vi "Create_Error.vi"(6 "Call chain":string[](array[string]), 7 "Restart text (\"\")":string, 8 "Status/Errors in":refnum<vi>, 9 "HiSPARC error":string, 10 "Warning? (false)":bool, 11 "Master?":T1) -> (0 "Status/Errors out":refnum<vi>)   [LabVIEW 2010]
doc: "Updates the Status/Errors-cluster with the message given by \"HiSPARC error\" together with the current time."
uses:
  Controls/Master.ctl
  Controls/Status_Errors_Elements.ctl
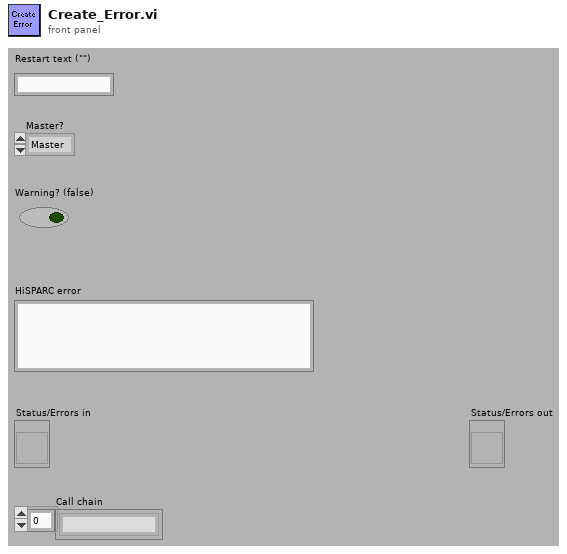
[diagram p1: front panel]
types:
  T1 = typedef "Master.ctl" = enum16{"Master", "Slave", "General"}
  T2 = typedef "Status_Errors_Elements.ctl" = enum16{"Default", "Errors", "Master status", "Slave status", "Master connected?", "Slave connected?", "Master GPS on board?", "Slave GPS on board?", "Master: slave detected?", "Slave: slave detected?", "Last message from master", "Last message from slave", "Master temperature"}
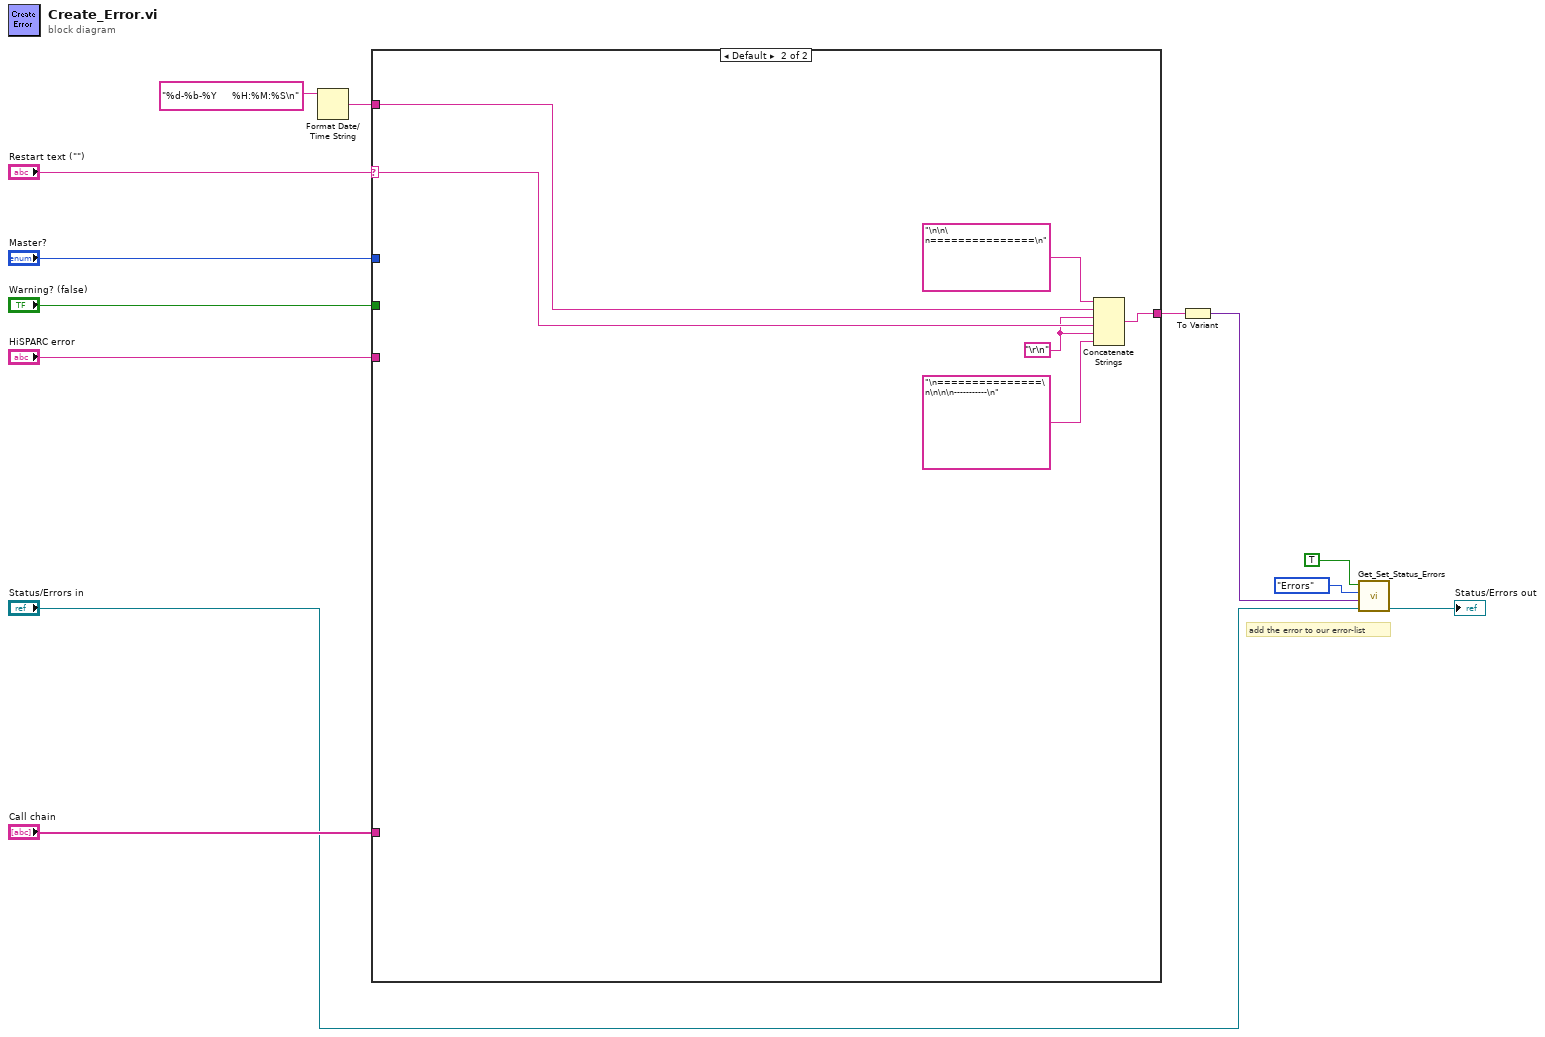
[diagram p0: block diagram]
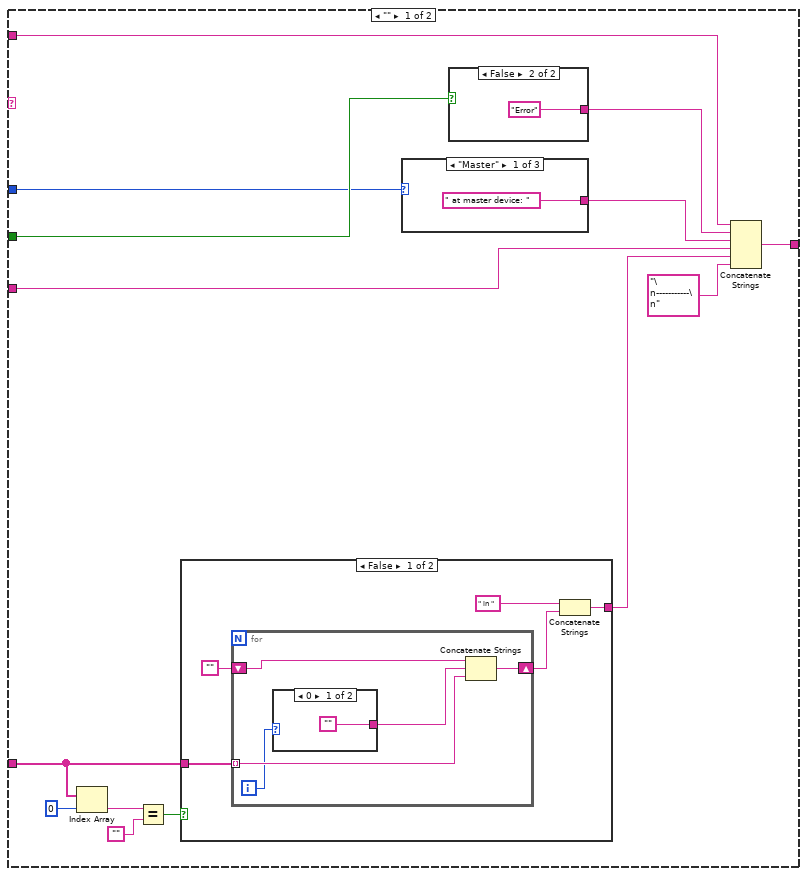
[diagram p2: hidden frame]
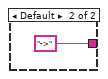
[diagram p3: hidden frame]
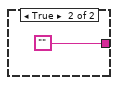
[diagram p4: hidden frame]
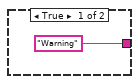
[diagram p5: hidden frame]
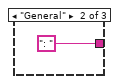
[diagram p6: hidden frame]
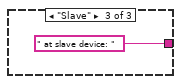
[diagram p7: hidden frame]
diagram:
  # "add the error to our error-list"
  n1 = Format Date/Time String(time format string (%c)="%d-%b-%Y     %H:%M:%S\n") -> (date/time string=w10:string)  [unwired: 2 out]
  n2 = case shown="Default" "Restart text (\"\")" {
    selector: "Restart text (\"\")" -> [_ w47]
    tunnel: "HiSPARC error" -> [w27 _]
    tunnel: "Warning? (false)" -> [w24 _]
    tunnel: w10 -> [w23 w51]
    tunnel: "Master?" -> [w21 _]
    tunnel: "Call chain" -> [w19 _]
    tunnel: [w14 w50] -> w4
    frame "" {
      n3 = Index Array(array=w19, index=0) -> (element=w17:string)
      n4 = Equal?(x=w17, y="") -> (x = y?=w15:bool)
      n5 = case shown="False" w15 {
        tunnel: [w29 ""] -> w20
        tunnel: w19 -> [w31 _]
        frame False {
          n6 = for {
            tunnel: w31 -> [w36] mode=indexing
            shift-right: [w37] -> w28
            shift-left: "" -> [w33]
            i -> [w35]
            n7 = case shown="0" w35 {
              tunnel: ["" "->"] -> w34
              frame 0 {
              }
              frame Default {
              }
            }
            n8 = Concatenate Strings(w33, w34, w36) -> (w37:string)
          }
          n9 = Concatenate Strings(" in ", w28) -> (w29:string)
        }
        frame True {
        }
      }
      n10 = case shown="\"Master\"" w21 {
        tunnel: [" at master device: " ("string") ": " ("string") " at slave device: " ("string")] -> w25
        frame "Master" {
        }
        frame "General" {
        }
        frame "Slave" {
        }
      }
      n11 = case shown="False" w24 {
        tunnel: ["Warning" ("string") "Error" ("string")] -> w22
        frame True {
        }
        frame False {
        }
      }
      n12 = Concatenate Strings(w23, w22, w25, w27, w20, "\n-----------\n") -> (w14:string)
    }
    frame Default {
      w46 = "\r\n"
      n13 = Concatenate Strings("\n\n\n===============\n", w51, w46, w47, w46, "\n===============\n\n\n\n-----------\n") -> (w50:string)
    }
  }
  n14 = To Variant(anything=w4) -> (Variant=w5:variant)
  n15 = call "Get_Set_Status_Errors.vi"("Status/Errors in"="Status/Errors in", "Value in"=w5, "Element"=Status_Errors_Elements."Errors", "Set?"=TRUE) -> ("Status/Errors out"=→"Status/Errors out":refnum<vi>)  [unwired: 7 out]
